vi "DIM_Read Sourcers.vi"(8 "error in (no error)":errorcluster, 11 "UI_Actor in":refnum<class "UI_Actor.lvclass">) -> (0 "error out":errorcluster, 2 "DIM Sourcers":string[](array[string]), 3 "UI_Actor out":refnum<class "UI_Actor.lvclass">)   [LabVIEW 2020, in "UI_Actor.lvlib" / "UI_Actor.lvclass"]
uses:
  UI_Actor.lvclass
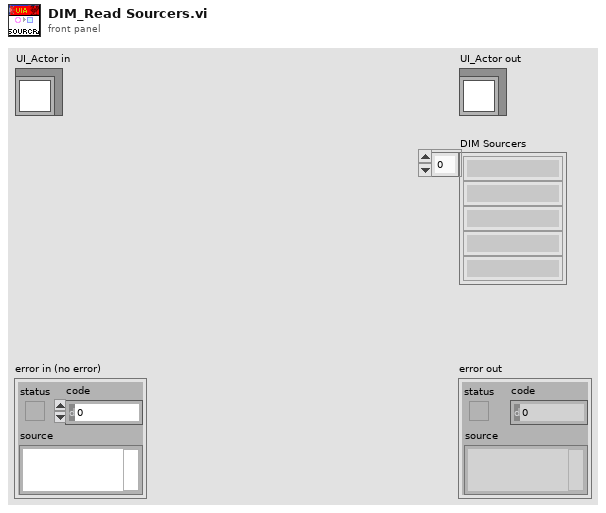
[diagram p1: front panel]
types:
  T1 = typedef "UI_Actor.lvlib/UI_Actor.lvclass/ctl_InternalMapItem.ctl" = cluster{"Config":refnum<class "Config.lvclass">, "LatestData":refnum<class "Data.lvclass">}
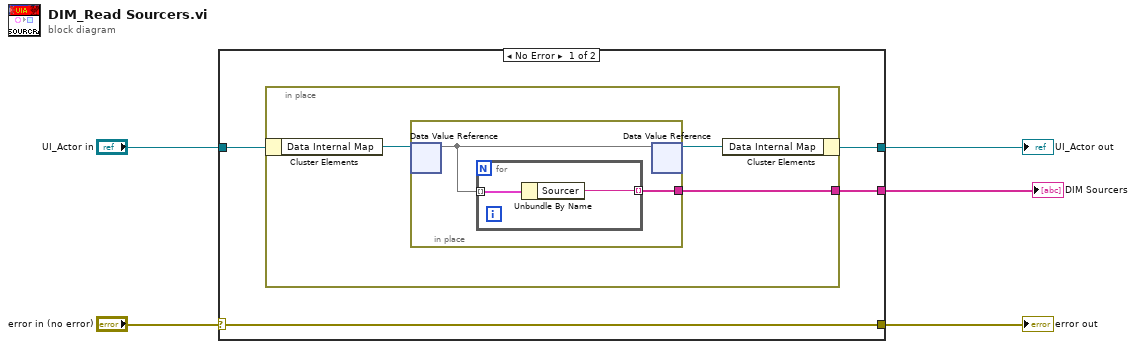
[diagram p0: block diagram]
diagram:
  n1 = case shown="No Error" "error in (no error)" {
    selector: "error in (no error)" -> [w9 w18]
    tunnel: [w9 w18] -> w4
    tunnel: [w7 w17] -> w2
    tunnel: "UI_Actor in" -> [w8 w17]
    tunnel: [w6 _] -> w1
    frame No Error {
      n2 = in-place {
        in-place-border: [w10] -> w6
        n3 = in-place-cluster #1(w8) -> ("Data Internal Map"=w12:refnum<data-value>)
        n4 = in-place {
          in-place-border: [w13] -> w10
          n5 = in-place-dvr #2(w12) -> (w14:map{string, map{string, T1}})  [unwired: 1 out]
          n6 = for {
            tunnel: w14 -> [w16] mode=indexing
            tunnel: [w15] -> w13 mode=indexing
            n7 = Unbundle By Name(w16) -> ("Sourcer"=w15:string)
          }
          n8 = in-place-dvr #2(w14) -> (w11:refnum<data-value>)  [unwired: 1 out]
        }
        n9 = in-place-cluster #1("Data Internal Map"=w11) -> (w7:refnum<class "UI_Actor.lvclass">)
      }
    }
    frame Error {
    }
  }
  "error out" <- w4
  "UI_Actor out" <- w2
  "DIM Sourcers" <- w1
